vi "Global 1.vi"() -> ()   [LabVIEW 2017]
panel:
  in  "Obj":i16
  in  "Data2":i16
  in  "Data1":i16
  out "V-Number":u8
  in  "TCNT":u64
  in  "Timer":i16
  in  "mode":i16
  in  "V-mode":i16
  out "V-Scale":sgl
  out "V-Ang":sgl
  out "V-y":sgl
  out "V-x":sgl
  in  "Vision":i16
  in  "led_counter":i8
  in  "loop":i16
  in  "Stop":bool=TRUE
  in  "Step":i16
  out "phi_ref":dbl
  out "Phi":dbl
  out "Y-ref":i64
  out "X-ref":i64
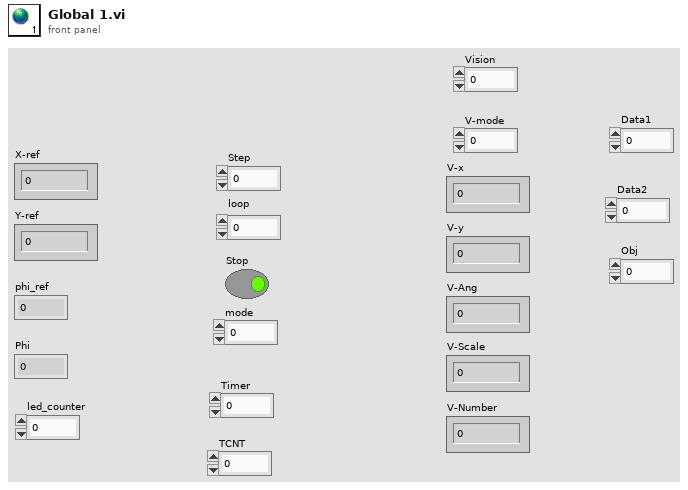
[diagram p1: front panel]
diagram:
